vi "OAT CIC Decimation.vi"(6 "initial state":cluster{"initial state":dbl[]}[](array[cluster]) {"initial state" format="%.2f"}, 7 "reset? (True)":bool=TRUE, 8 "error in (no error)":errorcluster, 10 "CIC filter settings":T1(array[cluster]), 11 "X":dbl[](array[numeric]) format="%.2f") -> (0 "error out":errorcluster, 3 "Y":dbl[](array[numeric]) format="%.2f", 4 "final state":cluster{"final state":dbl[]}[](array[cluster]) {"final state" format="%.2f"})   [LabVIEW 2017, in "SoundVib_Resampling.lvlib"]
uses:
  <vilib>/addons/Sound and Vibration/Order Analysis/Resample Order Tracking/SoundVib_Resampling.lvlib
  <resource>/sndvib.dll
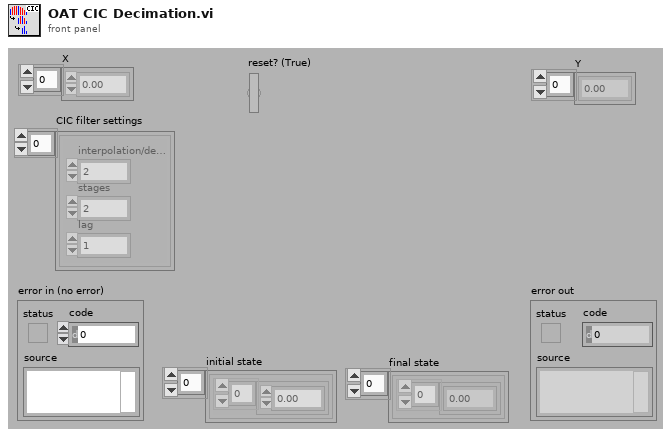
[diagram p1: front panel]
types:
  T1 = cluster{"interpolation/decimation factor":i32, "stages":i32, "lag":i32}[]
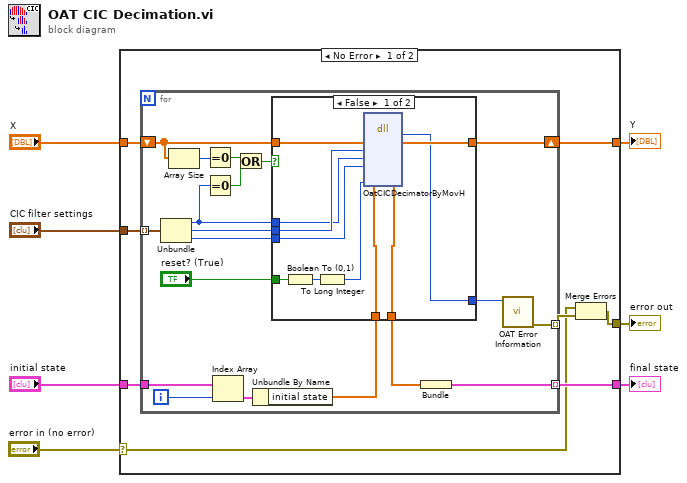
[diagram p0: block diagram]
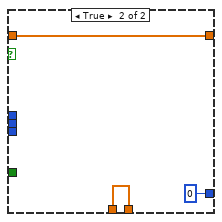
[diagram p2: hidden frame]
diagram:
  n1 = case shown="No Error" "error in (no error)" {
    selector: "error in (no error)" -> [w8 w50]
    tunnel: "CIC filter settings" -> [w15 _]
    tunnel: "X" -> [w14 w51]
    tunnel: [w13 w51] -> w5
    tunnel: "initial state" -> [w12 w49]
    tunnel: [w11 w49] -> w3
    tunnel: [w9 w50] -> w2
    frame No Error {
      n2 = for {
        tunnel: w15 -> [w34] mode=indexing
        shift-right: [w33] -> w13
        shift-left: w14 -> [w20]
        tunnel: w12 -> [w32]
        tunnel: [w24] -> w11 mode=indexing
        tunnel: [w22] -> w10 mode=indexing
        i -> [w31]
        n3 = Unbundle(w34) -> ("interpolation/decimation factor"=w27:i32, "stages"=w29:i32, "lag"=w28:i32)
        n4 = Array Size(array=w20) -> (size(s)=w19:i32)
        n5 = Equal To 0?(x=w19) -> (x = 0?=w18:bool)
        n6 = Equal To 0?(x=w27) -> (x = 0?=w17:bool)
        n7 = Index Array(array=w32, index=w31) -> (element=w30:cluster{"initial state":dbl[]})
        n8 = Or(x=w18, y=w17) -> (x .or. y?=w16:bool)
        n9 = Unbundle By Name(w30) -> ("initial state"=w26:dbl[])
        n10 = case shown="False" w16 {
          tunnel: w20 -> [w45 w48]
          tunnel: [w39 w48] -> w33
          tunnel: w29 -> [w44 _]
          tunnel: w28 -> [w43 _]
          tunnel: w27 -> [w42 _]
          tunnel: w26 -> [w41 w46]
          tunnel: [w40 w46] -> w25
          tunnel: [w38 0] -> w23
          tunnel: "reset? (True)" -> [w37 _]
          frame False {
            n11 = Boolean To (0,1)(Boolean=w37) -> (0, 1=w36:i16)
            n12 = To Long Integer(number=w36) -> (32bit integer=w35:i32)
            n13 = dll-call lib="C:/Program Files (x86)/National Instruments/LabVIEW 2017/resource/sndvib.*" fn="OatCICDecimatorByMovH"("xH"=w45, "stage"=w44, "dec_factor"=w42, "lag"=w43, "initH"=w41, "reset"=w35) -> ("return type"=w38:i32, "xH"=w39:dbl[], "initH"=w40:dbl[])  [unwired: 7 in, 2 out]
          }
          frame True {
          }
        }
        n14 = Bundle("initial state"=w25) -> (w24:cluster{"initial state":dbl[]})  [unwired: 1 in]
        n15 = call <vilib>:"OAT Error Information.vi"("error code"=w23) -> ("error out"=w22:errorcluster)  [unwired: 6 in]
      }
      n16 = Merge Errors(w8, w10) -> (w9:errorcluster)
    }
    frame Error {
    }
  }
  "Y" <- w5
  "final state" <- w3
  "error out" <- w2
